vi "ZMatrix2StatsCluster.vi"(11 "Array":dbl[][](array[numeric])) -> (3 "output cluster 2":T1 {"Mean |Z|" format="%#_6p"; "standard deviation |Z|" format="%#_6p"; "Mean Phase" format="%#_6p"; "standard deviation Phase" format="%#_6p"; "mean Ls" format="%#_6p"; "Standard dev. Ls" format="%#_6p"; "mean Real(Z)" format="%#_6p"; "Std. dev Real(Z)" format="%#_6p"; "mean Cs" format="%#_6p"; "Std. Dev. Cs" format="%#_6p"; "Mean Rp" format="%#_6p"; "Std. Dev. Rp" format="%#_6p"; "Mean Cp" format="%#_6p"; "Std. Dev. Cp" format="%#_6p"})   [LabVIEW 2022 SP3]
uses:
  <vilib>/Analysis/NI_AALBase.lvlib
panel:
  in  "output cluster":T1 {"Mean |Z|" format="%#_6p"; "standard deviation |Z|" format="%#_6p"; "Mean Phase" format="%#_6p"; "standard deviation Phase" format="%#_6p"; "mean Ls" format="%#_6p"; "Standard dev. Ls" format="%#_6p"; "mean Real(Z)" format="%#_6p"; "Std. dev Real(Z)" format="%#_6p"; "mean Cs" format="%#_6p"; "Std. Dev. Cs" format="%#_6p"; "Mean Rp" format="%#_6p"; "Std. Dev. Rp" format="%#_6p"; "Mean Cp" format="%#_6p"; "Std. Dev. Cp" format="%#_6p"}
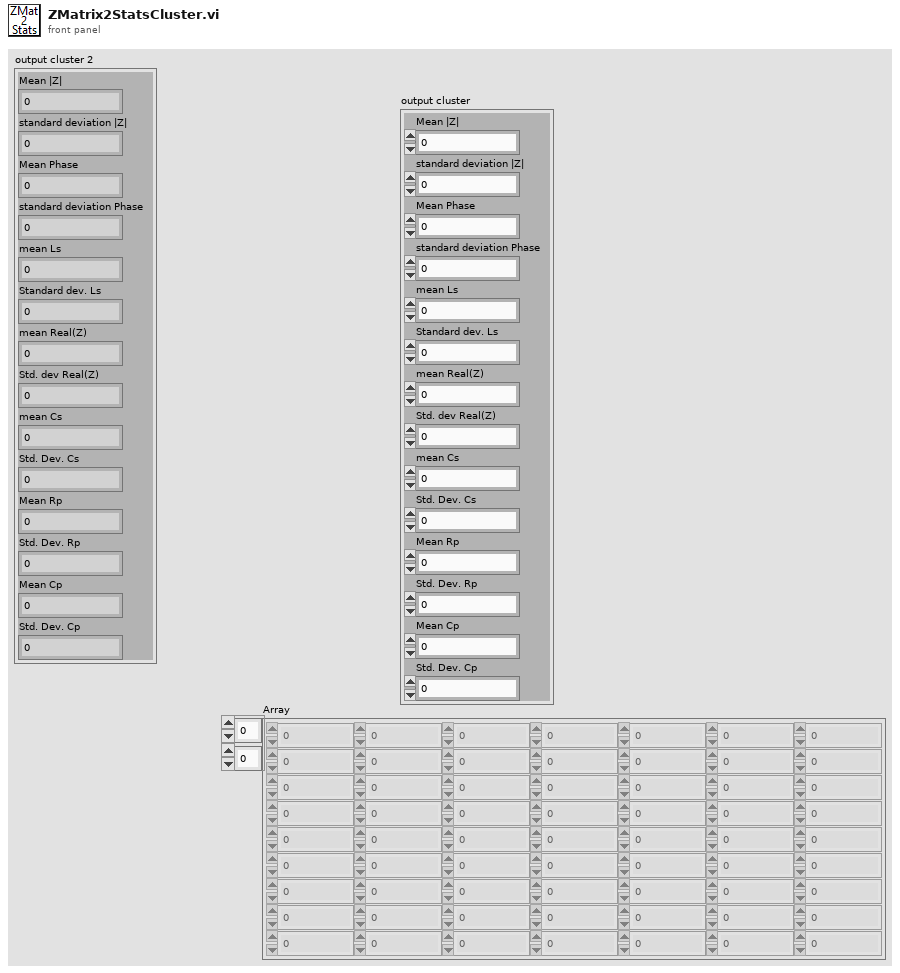
[diagram p1: front panel]
types:
  T1 = cluster{"Mean |Z|":dbl, "standard deviation |Z|":dbl, "Mean Phase":dbl, "standard deviation Phase":dbl, "mean Ls":dbl, "Standard dev. Ls":dbl, "mean Real(Z)":dbl, "Std. dev Real(Z)":dbl, "mean Cs":dbl, "Std. Dev. Cs":dbl, "Mean Rp":dbl, "Std. Dev. Rp":dbl, "Mean Cp":dbl, "Std. Dev. Cp":dbl}
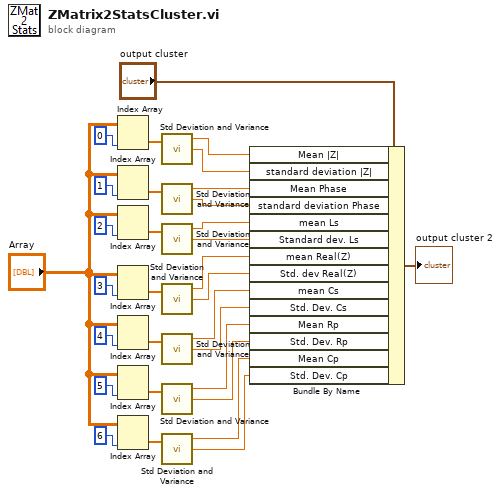
[diagram p0: block diagram]
diagram:
  n1 = Index Array(array="Array", index (col)=0 ("disabled index (col)")) -> (element=w28:dbl[])  [unwired: 1 in]
  n2 = Index Array(array="Array", index (col)=1 ("disabled index (col)")) -> (element=w25:dbl[])  [unwired: 1 in]
  n3 = Index Array(array="Array", index (col)=2 ("disabled index (col)")) -> (element=w21:dbl[])  [unwired: 1 in]
  n4 = Index Array(array="Array", index (col)=3 ("disabled index (col)")) -> (element=w17:dbl[])  [unwired: 1 in]
  n5 = Index Array(array="Array", index (col)=4 ("disabled index (col)")) -> (element=w13:dbl[])  [unwired: 1 in]
  n6 = Index Array(array="Array", index (col)=5 ("disabled index (col)")) -> (element=w9:dbl[])  [unwired: 1 in]
  n7 = Index Array(array="Array", index (col)=6 ("disabled index (col)")) -> (element=w5:dbl[])  [unwired: 1 in]
  n8 = call <vilib>:"Std Deviation and Variance.vi"("X"=w28) -> ("mean"=w27:dbl, "standard deviation"=w26:dbl)  [unwired: 1 in, 1 out]
  n9 = call <vilib>:"Std Deviation and Variance.vi"("X"=w25) -> ("mean"=w23:dbl, "standard deviation"=w22:dbl)  [unwired: 1 in, 1 out]
  n10 = call <vilib>:"Std Deviation and Variance.vi"("X"=w21) -> ("mean"=w19:dbl, "standard deviation"=w18:dbl)  [unwired: 1 in, 1 out]
  n11 = call <vilib>:"Std Deviation and Variance.vi"("X"=w17) -> ("mean"=w15:dbl, "standard deviation"=w14:dbl)  [unwired: 1 in, 1 out]
  n12 = call <vilib>:"Std Deviation and Variance.vi"("X"=w13) -> ("mean"=w11:dbl, "standard deviation"=w10:dbl)  [unwired: 1 in, 1 out]
  n13 = call <vilib>:"Std Deviation and Variance.vi"("X"=w9) -> ("mean"=w7:dbl, "standard deviation"=w6:dbl)  [unwired: 1 in, 1 out]
  n14 = call <vilib>:"Std Deviation and Variance.vi"("X"=w5) -> ("mean"=w3:dbl, "standard deviation"=w2:dbl)  [unwired: 1 in, 1 out]
  n15 = Bundle By Name(cluster="output cluster", "Mean |Z|"=w27, "standard deviation |Z|"=w26, "Mean Phase"=w23, "standard deviation Phase"=w22, "mean Ls"=w19, "Standard dev. Ls"=w18, "mean Real(Z)"=w15, "Std. dev Real(Z)"=w14, "mean Cs"=w11, "Std. Dev. Cs"=w10, "Mean Rp"=w7, "Std. Dev. Rp"=w6, "Mean Cp"=w3, "Std. Dev. Cp"=w2) -> (→"output cluster 2":T1)
